vi "DER Test.vi"(8 "error in":errorcluster, 11 "IED Test in":refnum<class "IED Test.lvclass">) -> (0 "error out":errorcluster, 2 "Test Result":T1=enum."Success", 3 "IED Test out":refnum<class "IED Test.lvclass">)   [LabVIEW 2018, in "IED Test Framework.lvlib" / "IED Test.lvclass"]
uses:
  IED Test.lvclass
  C:/Program Files (x86)/National Instruments/LabVIEW 2018/vi.lib/ActorFramework/Actor/Actor.lvclass
  C:/Users/Administrator/Desktop/2018LabVIEW EMS/EMS Generic Actor/EMS Generic/EMS Generic.lvclass
  Controls/Test Result.ctl
  DER Actor/DER/DER.lvclass
  C:/Users/Administrator/Desktop/2018LabVIEW EMS/IED Actors/Device DDS Communications Framework/Device DDS Communications/Device DDS Communications.lvclass
  <vilib>/ORNL/CSEISMIC DDS/CSEISMIC DDS Base/Data Types/Controls/DeviceClass Selector.ctl
  <vilib>/ORNL/CSEISMIC DDS/CSEISMIC DDS Base/CSEISMIC DDS.lvclass/CSEISMIC DDS.ctl
  <vilib>/ORNL/CSEISMIC DDS/CSEISMIC DDS Base/Data Types/Controls/DeviceID.ctl
  <vilib>/ActorFramework/Message Enqueuer/Message Enqueuer.lvclass/Message Enqueuer.ctl
  <vilib>/ORNL/CSEISMIC DDS/CSEISMIC DDS Base/Accessors/Write DDS Reference.vi
  <vilib>/ORNL/CSEISMIC DDS/CSEISMIC DDS Base/Accessors/Read DDS Reference.vi
  <vilib>/ActorFramework/Message Enqueuer/Enqueue.vi
  <vilib>/ORNL/CSEISMIC DDS/DDS Writer/DDS Writer.lvclass
  C:/Program Files (x86)/National Instruments/LabVIEW 2018/vi.lib/ORNL/CSEISMIC DDS/CSEISMIC DDS Base/CSEISMIC DDS.lvclass
  <vilib>/ActorFramework/Stop Msg/Stop Msg.lvclass
  C:/Program Files (x86)/National Instruments/LabVIEW 2018/vi.lib/ActorFramework/Message/Message.lvclass
  <vilib>/ORNL/CSEISMIC DDS/CSEISMIC DDS Base/Error Handler.vi
  <vilib>/ActorFramework/Message Priority Queue/Priority Enqueue.vi
  Device DDS Communications Framework/Device DDS Communications/Device DDS Communications.lvclass
  <vilib>/ActorFramework/Actor/Actor.lvclass
  <vilib>/ORNL/CSEISMIC DDS/CSEISMIC DDS Base/CSEISMIC DDS.lvclass
  EMS Generic Actor/EMS Generic/EMS Generic.lvclass
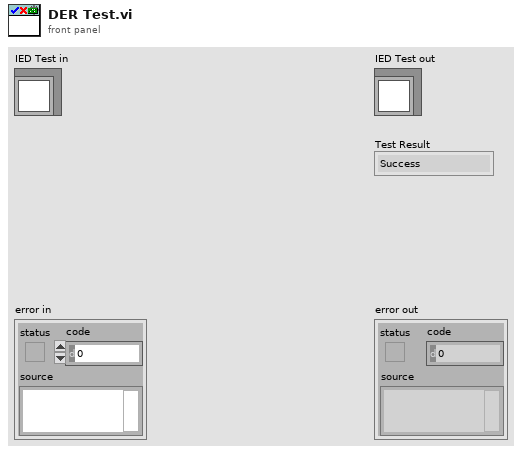
[diagram p1: front panel]
types:
  T1 = typedef "IED Test Framework.lvlib/IED Test.lvclass/Test Result.ctl" = enum16{"Invalid", "Success", "Failure", "Error", "Timeout"}
  T2 = typedef "CSEISMIC DDS.lvlib/CSEISMIC DDS.lvclass/DeviceID.ctl" = string
  T3 = typedef "CSEISMIC DDS.lvlib/CSEISMIC DDS.lvclass/DeviceClass Selector.ctl" = u16
  T4 = typedef "CSEISMIC DDS.lvlib/CSEISMIC DDS.lvclass/DER_Status.ctl" = cluster{"DeviceID":T2, "VFControl":bool, "PControl":bool, "QControl":bool, "PFControl":bool, "PVControl":bool, "Droop":bool, "Unbalanced":bool, "MicrogridVF":bool, "RealDroop(kW)":T5, "ReactiveDroop(kVar)":T5}
  T5 = typedef "CSEISMIC DDS.lvlib/CSEISMIC DDS.lvclass/DroopCurve.ctl" = cluster{"XMin":dbl, "XMax":dbl, "YMin":dbl, "YMax":dbl}
  T6 = typedef "CSEISMIC DDS.lvlib/CSEISMIC DDS.lvclass/DER_Info.ctl" = cluster{"DeviceID":T2, "LineConfig":u8[], "NominalVoltage(V)":dbl, "PowerRating(kVA)":dbl, "VFControl":bool, "PControl":bool, "QControl":bool, "PFControl":bool, "PVControl":bool, "Droop":bool, "DroopConfigurable":bool, "Unbalanced":bool}
  T7 = typedef "CSEISMIC DDS.lvlib/CSEISMIC DDS.lvclass/DER_Measurement.ctl" = cluster{"DeviceID":T2, "Voltage":dbl[], "Current":dbl[], "RealPower":dbl[], "ReactivePower":dbl[], "LineConfig":u8[], "Frequency":dbl}
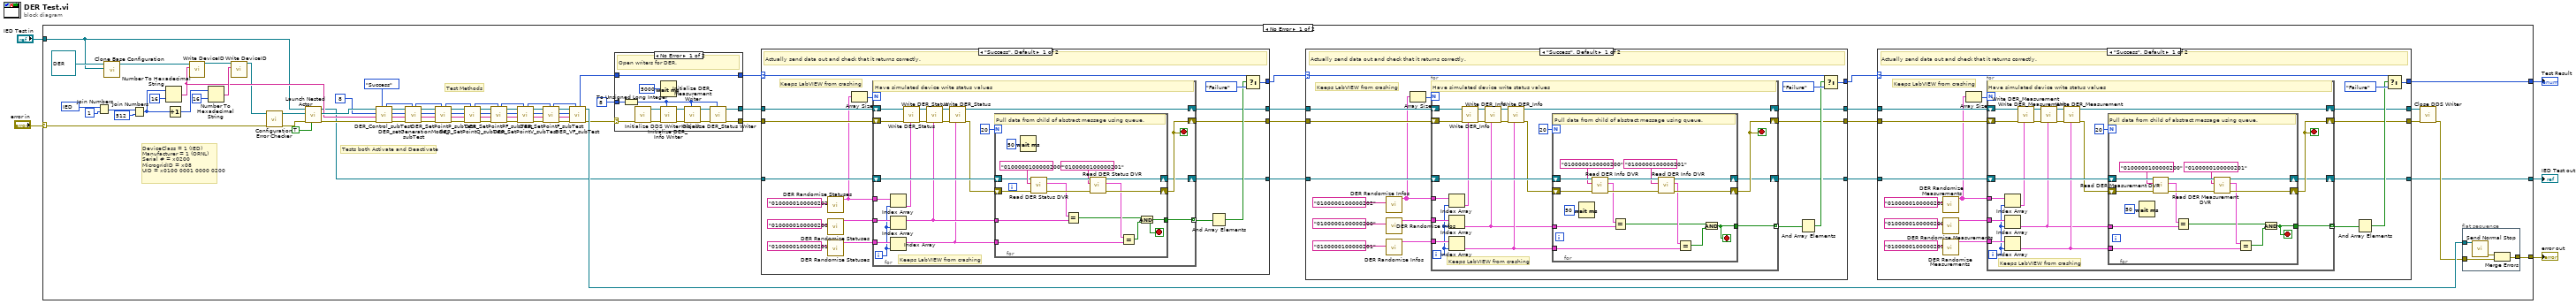
[diagram p0: block diagram]
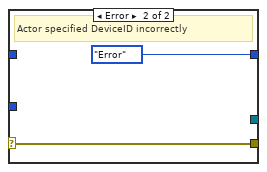
[diagram p5: hidden frame]
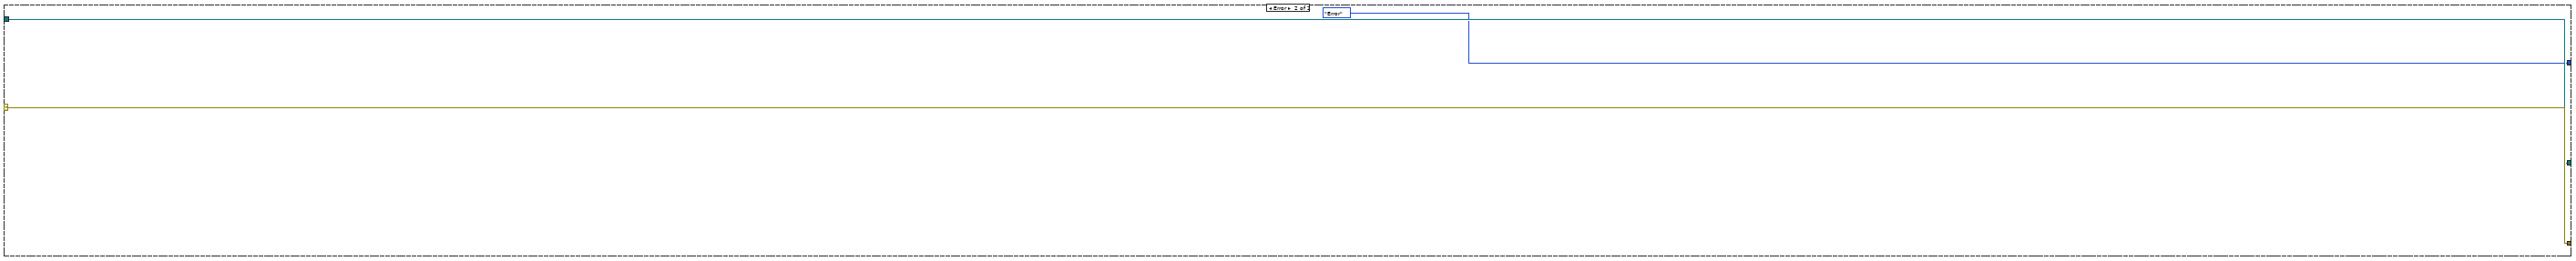
[diagram p6: hidden frame]
diagram:
  n1 = case shown="No Error" "error in" {
    selector: "error in" -> [w81 w281]
    tunnel: [w83 w281] -> w4
    tunnel: [w16 w280] -> w2
    tunnel: "IED Test in" -> [w20 w280]
    tunnel: [w27 Test_Result."Error" ("f")] -> w1
    frame No Error {
      w47 = T3 256 items=["Invalid"=0, "IED"=256, "DER"=512, "Relay"=768, "Meter"=1024, "Load"=1280, "Forecast"=1536, "Price"=1792, "Energy Storage"=513, "PV"=514, "Generator"=515, "Smart Relay"=769, "PCC"=770, "Smart Meter"=1025, "PMU"=1026, "HVAC"=1281] ("DeviceClass")
      # "Tests both Activate and Deactivate"
      # "Test Methods"
      # "DeviceClass = 1 (IED)\nManufacturer = 1 (ORNL)\nSerial # = x0200\nMicrogridID = x08\nUID = x0100 0001 0000 0200"
      n2 = Join Numbers(hi=w47, lo=u16 1 ("MicrogridID")) -> ((hi.lo)=w50:u32)
      n3 = call-dynamic "Clone Base Configuration.vi"("Source Object"=w20, "Target Object in"=refnum<class "DER.lvclass"> refnum ("DER Actor.lvlib:DER.lvclass")) -> ("Target Object out"=w22:refnum<class "DER.lvclass">)  [unwired: 9 in]
      n4 = Join Numbers(hi=w50, lo=u32 512 ("MicrogridID")) -> ((hi.lo)=w45:u64)
      n5 = Number To Hexadecimal String(1:i16 16 ("width (-)"), 2:w45) -> (0:w40:string)
      n6 = Increment(x=w45) -> (x+1=w43:u64)
      n7 = call-dynamic "Write DeviceID.vi"("DeviceID"=w40, "Device DDS Communications in"=w22) -> ("Device DDS Communications out"=w48:refnum<class "DER.lvclass">)  [unwired: 9 in]
      n8 = Number To Hexadecimal String(1:i16 16 ("width (-)"), 2:w43) -> (0:w42:string)
      n9 = call-dynamic "Write DeviceID.vi"("DeviceID"=w42, "Device DDS Communications in"=w48) -> ("Device DDS Communications out"=w23:refnum<class "DER.lvclass">)  [unwired: 9 in]
      n10 = call "Configuration Error Checker.vi"("error in"=w81, "Device DDS Communications in"=w23) -> ("error out"=w84:errorcluster, "Device DDS Communications out"=w82:refnum<class "DER.lvclass">)  [unwired: 8 in]
      n11 = call <vilib>:"Launch Nested Actor.vi"("Open Actor Core front panel? (F)"=TRUE, "error in (no error)"=w84, "Nested Actor"=w82, "Caller Actor in"=w20) -> ("error out"=w79:errorcluster, "Nested Actor's Enqueuer"=w80:refnum<class "Message Enqueuer.lvclass">, "Caller Actor out"=w17:refnum<class "IED Test.lvclass">)  [unwired: 5 in]
      n12 = call "DER_Control_subTest.vi"("Test Result in"=Test_Result."Success", "error in"=w79, "DeviceID"=w40, "MicrogridID"=u8 8, "Message Enqueuer in"=w80) -> ("error out"=w78:errorcluster, "dup DeviceID"=w73:T2, "dup MicrogridID"=w74:u8, "Message Enqueuer out"=w76:refnum<class "Message Enqueuer.lvclass">, "Test Result out"=w75:T1)  [unwired: 2 in]
      n13 = call "DER_setGenerationMode_subTest.vi"("Test Result in"=w75, "error in"=w78, "DeviceID"=w73, "MicrogridID"=w74, "Message Enqueuer in"=w76) -> ("error out"=w72:errorcluster, "dup DeviceID"=w69:T2, "dup MicrogridID"=w70:u8, "Message Enqueuer out"=w71:refnum<class "Message Enqueuer.lvclass">, "Test Result out"=w68:T1)  [unwired: 2 in]
      n14 = call "DER_SetPointP_subTest.vi"("Test Result in"=w68, "error in"=w72, "DeviceID"=w69, "MicrogridID"=w70, "Message Enqueuer in"=w71) -> ("error out"=w65:errorcluster, "dup DeviceID"=w63:T2, "dup MicrogridID"=w64:u8, "Message Enqueuer out"=w67:refnum<class "Message Enqueuer.lvclass">, "Test Result out"=w66:T1)  [unwired: 2 in]
      n15 = call "DER_SetPointQ_subTest.vi"("Test Result in"=w66, "error in"=w65, "DeviceID"=w63, "MicrogridID"=w64, "Message Enqueuer in"=w67) -> ("error out"=w60:errorcluster, "dup DeviceID"=w58:T2, "dup MicrogridID"=w59:u8, "Message Enqueuer out"=w62:refnum<class "Message Enqueuer.lvclass">, "Test Result out"=w61:T1)  [unwired: 2 in]
      n16 = call "DER_SetPointPF_subTest.vi"("Test Result in"=w61, "error in"=w60, "DeviceID"=w58, "MicrogridID"=w59, "Message Enqueuer in"=w62) -> ("error out"=w57:errorcluster, "dup DeviceID"=w53:T2, "dup MicrogridID"=w54:u8, "Message Enqueuer out"=w56:refnum<class "Message Enqueuer.lvclass">, "Test Result out"=w55:T1)  [unwired: 2 in]
      n17 = call "DER_SetPointV_subTest.vi"("Test Result in"=w55, "error in"=w57, "DeviceID"=w53, "MicrogridID"=w54, "Message Enqueuer in"=w56) -> ("error out"=w9:errorcluster, "dup DeviceID"=w8:T2, "dup MicrogridID"=w7:u8, "Message Enqueuer out"=w6:refnum<class "Message Enqueuer.lvclass">, "Test Result out"=w15:T1)  [unwired: 2 in]
      n18 = call "DER_SetPointF_subTest.vi"("Test Result in"=w15, "error in"=w9, "DeviceID"=w8, "MicrogridID"=w7, "Message Enqueuer in"=w6) -> ("error out"=w10:errorcluster, "dup DeviceID"=w11:T2, "dup MicrogridID"=w12:u8, "Message Enqueuer out"=w13:refnum<class "Message Enqueuer.lvclass">, "Test Result out"=w14:T1)  [unwired: 2 in]
      n19 = call "DER_VF_subTest.vi"("Test Result in"=w14, "error in"=w10, "DeviceID"=w11, "MicrogridID"=w12, "Message Enqueuer in"=w13) -> ("error out"=w39:errorcluster, "Message Enqueuer out"=w52:refnum<class "Message Enqueuer.lvclass">, "Test Result out"=w34:T1)  [unwired: 2 in, 2 out]
      n20 = case shown="No Error" w39 {
        selector: w39 -> [w274 w278]
        tunnel: [w265 w278] -> w36
        tunnel: u32 8 ("domain id") -> [w276 _]
        tunnel: [w266 _] -> w37
        tunnel: [w271 Test_Result."Error" ("Test Result")] -> w35
        tunnel: w34 -> [w271 _]
        frame No Error {
          # "Open writers for DER."
          n21 = To Unsigned Long Integer(number=w276) -> (unsigned 32bit integer=w264:u32)
          n22 = call <vilib>:"Initialize DDS Writer Object.vi"("error in"=w274) -> ("error out"=w273:errorcluster, "DDS Writer out"=w272:refnum<class "DDS Writer.lvclass">)  [unwired: 9 in]
          n23 = Wait (ms)(milliseconds to wait=u32 5000) -> ()  [unwired: 1 out]
          n24 = call <vilib>:"Initialize DER_Info Writer.vi"("MicrogridID"=w264, "error in"=w273, "DDS Writer in"=w272) -> ("error out"=w269:errorcluster, "DDS Writer out"=w270:refnum<class "DDS Writer.lvclass">)  [unwired: 7 in]
          n25 = call <vilib>:"Initialize DER_Measurement Writer.vi"("MicrogridID"=w264, "error in"=w269, "DDS Writer in"=w270) -> ("error out"=w268:errorcluster, "DDS Writer"=w267:refnum<class "DDS Writer.lvclass">)  [unwired: 7 in]
          n26 = call <vilib>:"Initialize DER_Status Writer.vi"("MicrogridID"=w264, "error in"=w268, "DDS Writer in"=w267) -> ("error out"=w265:errorcluster, "DDS Writer out"=w266:refnum<class "DDS Writer.lvclass">)  [unwired: 7 in]
        }
        frame Error {
          # "Actor specified DeviceID incorrectly"
        }
      }
      n27 = case shown="\"Success\", Default" w35 {
        selector: w35 -> [w222 w262]
        tunnel: w37 -> [w223 w261]
        tunnel: w17 -> [w217 w260]
        tunnel: w36 -> [w218 w263]
        tunnel: [w220 w262] -> w31
        tunnel: [w216 w263] -> w32
        tunnel: [w213 w261] -> w33
        tunnel: [w206 w260] -> w18
        frame "Success", Default {
          # "Keeps LabVIEW from crashing"
          # "Actually send data out and check that it returns correctly."
          n28 = call "DER Randomize Statuses.vi"("DeviceID"=T2 "0100000100000202" ("(hi.lo)")) -> ("DER_Status Array out"=w211:T4[])  [unwired: 10 in]
          n29 = call "DER Randomize Statuses.vi"("DeviceID"=T2 "0100000100000200" ("(hi.lo)")) -> ("DER_Status Array out"=w209:T4[])  [unwired: 10 in]
          n30 = call "DER Randomize Statuses.vi"("DeviceID"=T2 "0100000100000201" ("(hi.lo)")) -> ("DER_Status Array out"=w207:T4[])  [unwired: 10 in]
          n31 = Array Size(array=w211) -> (size(s)=w214:i32)
          n32 = for {
            N: w214 -> [_]
            shift-right: [w240] -> w213
            shift-left: w223 -> [w243]
            tunnel: w211 -> [w236]
            tunnel: w207 -> [w231]
            tunnel: w209 -> [w232]
            shift-right: [w233] -> w216
            shift-left: w218 -> [w239]
            tunnel: [w225] -> w215 mode=indexing
            shift-right: [w224] -> w206
            shift-left: w217 -> [w235]
            i -> [w229]
            stop <- w233 stop-if-true
            # "Keeps LabVIEW from crashing"
            # "Have simulated device write status values"
            n33 = Index Array(array=w236, index=w229) -> (element=w228:T4)
            n34 = Index Array(array=w232, index=w229) -> (element=w227:T4)
            n35 = Index Array(array=w231, index=w229) -> (element=w226:T4)
            n36 = call <vilib>:"Write DER_Status.vi"("DER_Status"=w228, "error in"=w239, "DDS Writer in"=w243) -> ("error out"=w238:errorcluster, "DDS Writer out"=w242:refnum<class "DDS Writer.lvclass">)  [unwired: 7 in]
            n37 = call <vilib>:"Write DER_Status.vi"("DER_Status"=w227, "error in"=w238, "DDS Writer in"=w242) -> ("error out"=w237:errorcluster, "DDS Writer out"=w241:refnum<class "DDS Writer.lvclass">)  [unwired: 7 in]
            n38 = call <vilib>:"Write DER_Status.vi"("DER_Status"=w226, "error in"=w237, "DDS Writer in"=w241) -> ("error out"=w234:errorcluster, "DDS Writer out"=w240:refnum<class "DDS Writer.lvclass">)  [unwired: 7 in]
            n39 = for {
              N: 20 -> [_]
              shift-right: [w254] -> w233
              shift-left: w234 -> [w257]
              tunnel: w227 -> [w251]
              tunnel: w226 -> [w249]
              tunnel: [w245] -> w225
              shift-right: [w244] -> w224
              shift-left: w235 -> [w258]
              stop <- w245 stop-if-true
              # "Pull data from child of abstract message using queue."
              n40 = Wait (ms)(milliseconds to wait=u32 50) -> ()  [unwired: 1 out]
              n41 = call "Read DER Status DVR.vi"("error in"=w257, "DeviceID"=T2 "0100000100000200" ("(hi.lo)"), "EMS Generic in"=w258) -> ("error out"=w256:errorcluster, "DER_Status"=w250:T4, "EMS Generic out"=w255:refnum<class "IED Test.lvclass">)  [unwired: 5 in, 1 out]
              n42 = Equal?(x=w250, y=w251) -> (x = y?=w246:bool)
              n43 = call "Read DER Status DVR.vi"("error in"=w256, "DeviceID"=T2 "0100000100000201" ("(hi.lo)"), "EMS Generic in"=w255) -> ("error out"=w254:errorcluster, "DER_Status"=w248:T4, "EMS Generic out"=w244:refnum<class "IED Test.lvclass">)  [unwired: 5 in, 1 out]
              n44 = Equal?(x=w248, y=w249) -> (x = y?=w247:bool)
              n45 = And(x=w246, y=w247) -> (x .and. y?=w245:bool)
            }
          }
          n46 = And Array Elements(Boolean array=w215) -> (logical AND=w219:bool)
          n47 = Select(t=w222, s=w219, f=Test_Result."Failure") -> (s? t:f=w220:T1)
        }
        frame "Error" {
        }
      }
      n48 = case shown="\"Success\", Default" w31 {
        selector: w31 -> [w164 w204]
        tunnel: w33 -> [w165 w203]
        tunnel: w18 -> [w159 w202]
        tunnel: w32 -> [w160 w205]
        tunnel: [w162 w204] -> w30
        tunnel: [w158 w205] -> w28
        tunnel: [w156 w203] -> w29
        tunnel: [w148 w202] -> w19
        frame "Success", Default {
          # "Keeps LabVIEW from crashing"
          # "Actually send data out and check that it returns correctly."
          n49 = call "DER Randomize Infos.vi"("DeviceID"=T2 "0100000100000202" ("(hi.lo)")) -> ("DER Info Array"=w154:T6[])  [unwired: 10 in]
          n50 = call "DER Randomize Infos.vi"("DeviceID"=T2 "0100000100000200" ("(hi.lo)")) -> ("DER Info Array"=w152:T6[])  [unwired: 10 in]
          n51 = call "DER Randomize Infos.vi"("DeviceID"=T2 "0100000100000201" ("(hi.lo)")) -> ("DER Info Array"=w150:T6[])  [unwired: 10 in]
          n52 = Array Size(array=w154) -> (size(s)=w157:i32)
          n53 = for {
            N: w157 -> [_]
            shift-right: [w182] -> w156
            shift-left: w165 -> [w185]
            tunnel: w154 -> [w178]
            tunnel: w150 -> [w173]
            tunnel: w152 -> [w174]
            shift-right: [w175] -> w158
            shift-left: w160 -> [w181]
            tunnel: [w167] -> w149 mode=indexing
            shift-right: [w166] -> w148
            shift-left: w159 -> [w177]
            i -> [w171]
            stop <- w175 stop-if-true
            # "Keeps LabVIEW from crashing"
            # "Have simulated device write status values"
            n54 = Index Array(array=w178, index=w171) -> (element=w170:T6)
            n55 = Index Array(array=w174, index=w171) -> (element=w168:T6)
            n56 = Index Array(array=w173, index=w171) -> (element=w169:T6)
            n57 = call <vilib>:"Write DER_Info.vi"("DER_Info"=w170, "error in"=w181, "DDS Writer in"=w185) -> ("error out"=w180:errorcluster, "DDS Writer out"=w184:refnum<class "DDS Writer.lvclass">)  [unwired: 7 in]
            n58 = call <vilib>:"Write DER_Info.vi"("DER_Info"=w168, "error in"=w180, "DDS Writer in"=w184) -> ("error out"=w179:errorcluster, "DDS Writer out"=w183:refnum<class "DDS Writer.lvclass">)  [unwired: 7 in]
            n59 = call <vilib>:"Write DER_Info.vi"("DER_Info"=w169, "error in"=w179, "DDS Writer in"=w183) -> ("error out"=w176:errorcluster, "DDS Writer out"=w182:refnum<class "DDS Writer.lvclass">)  [unwired: 7 in]
            n60 = for {
              N: 20 -> [_]
              shift-right: [w194] -> w175
              shift-left: w176 -> [w200]
              tunnel: w169 -> [w191]
              tunnel: w168 -> [w192]
              tunnel: [w187] -> w167
              shift-right: [w186] -> w166
              shift-left: w177 -> [w199]
              stop <- w187 stop-if-true
              # "Pull data from child of abstract message using queue."
              n61 = Wait (ms)(milliseconds to wait=u32 50) -> ()  [unwired: 1 out]
              n62 = call "Read DER Info DVR.vi"("error in"=w200, "DeviceID"=T2 "0100000100000200" ("(hi.lo)"), "EMS Generic in"=w199) -> ("error out"=w198:errorcluster, "DER_Info"=w193:T6, "EMS Generic out"=w197:refnum<class "IED Test.lvclass">)  [unwired: 5 in, 1 out]
              n63 = Equal?(x=w193, y=w192) -> (x = y?=w188:bool)
              n64 = call "Read DER Info DVR.vi"("error in"=w198, "DeviceID"=T2 "0100000100000201" ("(hi.lo)"), "EMS Generic in"=w197) -> ("error out"=w194:errorcluster, "DER_Info"=w190:T6, "EMS Generic out"=w186:refnum<class "IED Test.lvclass">)  [unwired: 5 in, 1 out]
              n65 = Equal?(x=w190, y=w191) -> (x = y?=w189:bool)
              n66 = And(x=w188, y=w189) -> (x .and. y?=w187:bool)
            }
          }
          n67 = And Array Elements(Boolean array=w149) -> (logical AND=w161:bool)
          n68 = Select(t=w164, s=w161, f=Test_Result."Failure") -> (s? t:f=w162:T1)
        }
        frame "Error" {
        }
      }
      n69 = case shown="\"Success\", Default" w30 {
        selector: w30 -> [w106 w146]
        tunnel: w29 -> [w107 w145]
        tunnel: w19 -> [w101 w144]
        tunnel: w28 -> [w102 w147]
        tunnel: [w104 w146] -> w27
        tunnel: [w100 w147] -> w26
        tunnel: [w98 w145] -> w25
        tunnel: [w90 w144] -> w16
        frame "Success", Default {
          # "Keeps LabVIEW from crashing"
          # "Actually send data out and check that it returns correctly."
          n70 = call "DER Randomize Measurements.vi"("DeviceID"=T2 "0100000100000202" ("(hi.lo)")) -> ("DER Measurement Array"=w96:T7[])  [unwired: 10 in]
          n71 = call "DER Randomize Measurements.vi"("DeviceID"=T2 "0100000100000200" ("(hi.lo)")) -> ("DER Measurement Array"=w94:T7[])  [unwired: 10 in]
          n72 = call "DER Randomize Measurements.vi"("DeviceID"=T2 "0100000100000201" ("(hi.lo)")) -> ("DER Measurement Array"=w92:T7[])  [unwired: 10 in]
          n73 = Array Size(array=w96) -> (size(s)=w99:i32)
          n74 = for {
            N: w99 -> [_]
            shift-right: [w124] -> w98
            shift-left: w107 -> [w127]
            tunnel: w96 -> [w120]
            tunnel: w92 -> [w115]
            tunnel: w94 -> [w116]
            shift-right: [w117] -> w100
            shift-left: w102 -> [w123]
            tunnel: [w109] -> w91 mode=indexing
            shift-right: [w108] -> w90
            shift-left: w101 -> [w119]
            i -> [w113]
            stop <- w117 stop-if-true
            # "Keeps LabVIEW from crashing"
            # "Have simulated device write status values"
            n75 = Index Array(array=w120, index=w113) -> (element=w112:T7)
            n76 = Index Array(array=w116, index=w113) -> (element=w110:T7)
            n77 = Index Array(array=w115, index=w113) -> (element=w111:T7)
            n78 = call <vilib>:"Write DER_Measurement.vi"("DER_Measurement"=w112, "error in"=w123, "DDS Writer in"=w127) -> ("error out"=w122:errorcluster, "DDS Writer out"=w126:refnum<class "DDS Writer.lvclass">)  [unwired: 7 in]
            n79 = call <vilib>:"Write DER_Measurement.vi"("DER_Measurement"=w110, "error in"=w122, "DDS Writer in"=w126) -> ("error out"=w121:errorcluster, "DDS Writer out"=w125:refnum<class "DDS Writer.lvclass">)  [unwired: 7 in]
            n80 = call <vilib>:"Write DER_Measurement.vi"("DER_Measurement"=w111, "error in"=w121, "DDS Writer in"=w125) -> ("error out"=w118:errorcluster, "DDS Writer out"=w124:refnum<class "DDS Writer.lvclass">)  [unwired: 7 in]
            n81 = for {
              N: 20 -> [_]
              shift-right: [w137] -> w117
              shift-left: w118 -> [w142]
              tunnel: w111 -> [w133]
              tunnel: w110 -> [w135]
              tunnel: [w129] -> w109
              shift-right: [w128] -> w108
              shift-left: w119 -> [w141]
              stop <- w129 stop-if-true
              # "Pull data from child of abstract message using queue."
              n82 = Wait (ms)(milliseconds to wait=u32 50) -> ()  [unwired: 1 out]
              n83 = call "Read DER Measurement DVR.vi"("error in"=w142, "DeviceID"=T2 "0100000100000200" ("(hi.lo)"), "EMS Generic in"=w141) -> ("error out"=w138:errorcluster, "DER_Measurement"=w134:T7, "EMS Generic out"=w139:refnum<class "IED Test.lvclass">)  [unwired: 5 in, 1 out]
              n84 = Equal?(x=w134, y=w135) -> (x = y?=w131:bool)
              n85 = call "Read DER Measurement DVR.vi"("error in"=w138, "DeviceID"=T2 "0100000100000201" ("(hi.lo)"), "EMS Generic in"=w139) -> ("error out"=w137:errorcluster, "DER_Measurement"=w132:T7, "EMS Generic out"=w128:refnum<class "IED Test.lvclass">)  [unwired: 5 in, 1 out]
              n86 = Equal?(x=w132, y=w133) -> (x = y?=w130:bool)
              n87 = And(x=w131, y=w130) -> (x .and. y?=w129:bool)
            }
          }
          n88 = And Array Elements(Boolean array=w91) -> (logical AND=w103:bool)
          n89 = Select(t=w106, s=w103, f=Test_Result."Failure") -> (s? t:f=w104:T1)
        }
        frame "Error" {
        }
      }
      n90 = call <vilib>:"Close DDS Writer.vi"("error in"=w26, "DDS Writer in"=w25) -> ("error out"=w24:errorcluster)  [unwired: 9 in]
      n91 = flat-sequence {
        tunnel: w52 -> [w89]
        tunnel: [w87] -> w83
        tunnel: w24 -> [w86]
        frame #0 {
          n92 = call <vilib>:"Send Normal Stop.vi"("Message Enqueuer"=w89) -> ("error out"=w88:errorcluster)  [unwired: 10 in]
          n93 = Merge Errors(w88, w86) -> (w87:errorcluster)
        }
      }
    }
    frame Error {
    }
  }
  "error out" <- w4
  "IED Test out" <- w2
  "Test Result" <- w1
